vi "SubVI_Send_Impedance_Values.vi"(8 "error in (no error)":errorcluster, 11 "Raw Impedances In":T1) -> (0 "error out":errorcluster)   [LabVIEW 2020]
uses:
  <extravilib>/ChannelInstances/Lossy Stream-a[.,.](dbl)/)Channel.ctl
  <extravilib>/ChannelInstances/Lossy Stream-a[.,.](dbl)/EndpointRead.vi
  Global 1.vi
  <extravilib>/ChannelInstances/Lossy Stream-a[.,.](dbl)/)Channel.vi
  <resource>/ChannelSupport/_ChannelSupport/WaitIfNeeded.vi
  <extravilib>/ChannelInstances/Lossy Stream-a[.,.](dbl).lvlib
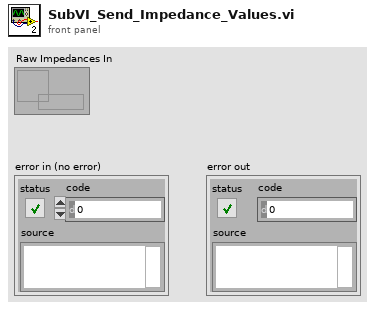
[diagram p1: front panel]
types:
  T1 = typedef "Lossy Stream-a[.,.](dbl).lvlib/)Channel.ctl" = refnum<queue>
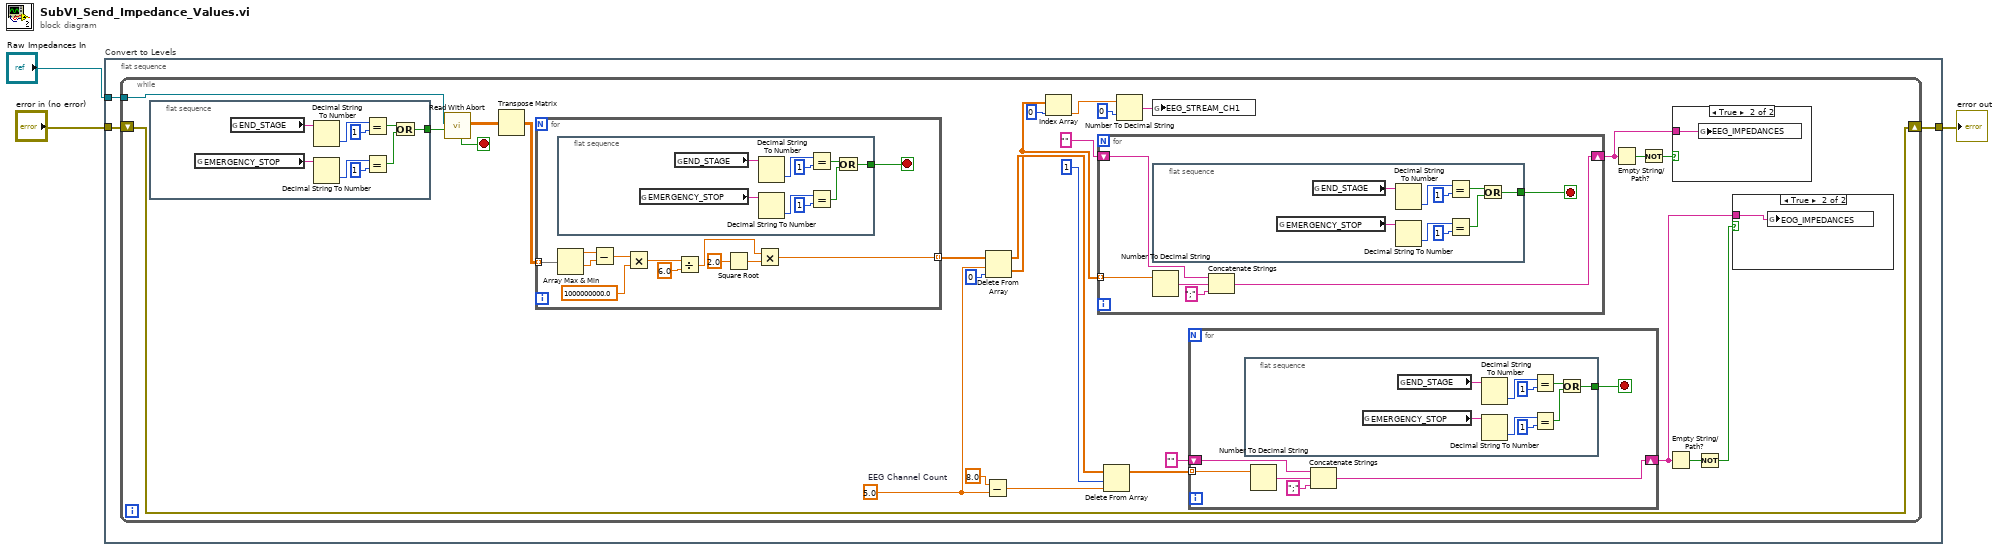
[diagram p0: block diagram]
diagram:
  n1 = flat-sequence "Convert to Levels" {
    tunnel: "Raw Impedances In" -> [w6]
    tunnel: [w5] -> w2
    tunnel: "error in (no error)" -> [w4]
    frame #0 {
      n2 = while {
        tunnel: w6 -> [w33]
        shift-right: [w29] -> w5
        shift-left: w4 -> [w29]
        stop <- w32 stop-if-true
        w18 = 5.0  # EEG Channel Count
        n3 = flat-sequence {
          tunnel: [w36] -> w13
          frame #0 {
            n4 = global read "Global 1.vi" "EMERGENCY_STOP"() -> (w39:string)
            n5 = global read "Global 1.vi" "END_STAGE"() -> (w44:string)
            n6 = Decimal String To Number(string=w44) -> (number=w43:i32)  [unwired: 2 in, 1 out]
            n7 = Decimal String To Number(string=w39) -> (number=w41:i32)  [unwired: 2 in, 1 out]
            n8 = Equal?(x=w43, y=1) -> (x = y?=w37:bool)
            n9 = Equal?(x=w41, y=1) -> (x = y?=w38:bool)
            n10 = Or(x=w37, y=w38) -> (x .or. y?=w36:bool)
          }
        }
        n11 = call <extravilib>:"Read With Abort.vi"("abort"=w13, "channel"=w33) -> ("element"=w28:dbl[][], "aborted?"=w32:bool)  [unwired: 3 in, 5 out]
        n12 = Transpose Matrix(1:w28) -> (0:w27:dbl[][])
        n13 = for {
          tunnel: w27 -> [w86] mode=indexing
          tunnel: [w76] -> w26 mode=indexing
          stop <- w75 stop-if-true
          n14 = flat-sequence {
            tunnel: [w87] -> w75
            frame #0 {
              n15 = global read "Global 1.vi" "EMERGENCY_STOP"() -> (w90:string)
              n16 = global read "Global 1.vi" "END_STAGE"() -> (w95:string)
              n17 = Decimal String To Number(string=w95) -> (number=w94:i32)  [unwired: 2 in, 1 out]
              n18 = Decimal String To Number(string=w90) -> (number=w92:i32)  [unwired: 2 in, 1 out]
              n19 = Equal?(x=w94, y=1) -> (x = y?=w88:bool)
              n20 = Equal?(x=w92, y=1) -> (x = y?=w89:bool)
              n21 = Or(x=w88, y=w89) -> (x .or. y?=w87:bool)
            }
          }
          n22 = Array Max & Min ("Max & Min")(array=w86) -> (max value=w79:dbl, min value=w78:dbl)  [unwired: 2 out]
          n23 = Subtract(x=w79, y=w78) -> (x-y=w77:dbl)
          n24 = Multiply(x=w77, y=1000000000.0) -> (x*y=w84:dbl)
          n25 = Divide(x=w84, y=6.0) -> (x/y=w82:dbl)
          n26 = Square Root(x=2.0) -> (sqrt(x)=w80:dbl)
          n27 = Multiply(x=w82, y=w80) -> (x*y=w76:dbl)
        }
        n28 = Subtract(x=8.0, y=w18) -> (x-y=w23:dbl)
        n29 = Delete From Array(array=w26, length=w18, index=0) -> (deleted portion=w14:dbl[], array with subset deleted=w31:dbl[])
        n30 = Index Array(array=w14, index=0) -> (element=w20:dbl)
        n31 = for {
          tunnel: w14 -> [w61] mode=indexing
          shift-right: [w63] -> w12
          shift-left: "" -> [w62]
          stop <- w60 stop-if-true
          n32 = flat-sequence {
            tunnel: [w66] -> w60
            frame #0 {
              n33 = global read "Global 1.vi" "EMERGENCY_STOP"() -> (w69:string)
              n34 = global read "Global 1.vi" "END_STAGE"() -> (w74:string)
              n35 = Decimal String To Number(string=w74) -> (number=w73:i32)  [unwired: 2 in, 1 out]
              n36 = Decimal String To Number(string=w69) -> (number=w71:i32)  [unwired: 2 in, 1 out]
              n37 = Equal?(x=w73, y=1) -> (x = y?=w67:bool)
              n38 = Equal?(x=w71, y=1) -> (x = y?=w68:bool)
              n39 = Or(x=w67, y=w68) -> (x .or. y?=w66:bool)
            }
          }
          n40 = Number To Decimal String(number=w61) -> (decimal integer string=w65:string)  [unwired: 1 in]
          n41 = Concatenate Strings(w62, w65, ";" ("string")) -> (w63:string)
        }
        n42 = Delete From Array(array=w31, length=1, index=w23) -> (array with subset deleted=w15:dbl[])  [unwired: 1 out]
        n43 = Number To Decimal String(number=w20, width (-)=i16 0) -> (decimal integer string=w19:string)
        n44 = global write "Global 1.vi" "EEG_STREAM_CH1"(w19) -> ()
        n45 = for {
          tunnel: w15 -> [w46] mode=indexing
          shift-right: [w48] -> w8
          shift-left: "" -> [w47]
          stop <- w45 stop-if-true
          n46 = flat-sequence {
            tunnel: [w51] -> w45
            frame #0 {
              n47 = global read "Global 1.vi" "EMERGENCY_STOP"() -> (w54:string)
              n48 = global read "Global 1.vi" "END_STAGE"() -> (w59:string)
              n49 = Decimal String To Number(string=w59) -> (number=w58:i32)  [unwired: 2 in, 1 out]
              n50 = Decimal String To Number(string=w54) -> (number=w56:i32)  [unwired: 2 in, 1 out]
              n51 = Equal?(x=w58, y=1) -> (x = y?=w52:bool)
              n52 = Equal?(x=w56, y=1) -> (x = y?=w53:bool)
              n53 = Or(x=w52, y=w53) -> (x .or. y?=w51:bool)
            }
          }
          n54 = Number To Decimal String(number=w46) -> (decimal integer string=w50:string)  [unwired: 1 in]
          n55 = Concatenate Strings(w47, w50, ";" ("string")) -> (w48:string)
        }
        n56 = Empty String/Path?(string/path=w12) -> (empty?=w11:bool)
        n57 = Not(x=w11) -> (.not. x?=w10:bool)
        n58 = Empty String/Path?(string/path=w8) -> (empty?=w9:bool)
        n59 = case shown="True" w10 {
          tunnel: w12 -> [_ w35]
          frame False {
          }
          frame True {
            n60 = global write "Global 1.vi" "EEG_IMPEDANCES"(w35) -> ()
          }
        }
        n61 = Not(x=w9) -> (.not. x?=w7:bool)
        n62 = case shown="True" w7 {
          tunnel: w8 -> [_ w34]
          frame False {
          }
          frame True {
            n63 = global write "Global 1.vi" "EOG_IMPEDANCES"(w34) -> ()
          }
        }
      }
    }
  }
  "error out" <- w2
